vi "extraeIO.vi"(8 "error in TCP":errorcluster, 10 "path":path, 11 "connection IDin":refnum<k5>) -> (0 "error out TCP":errorcluster, 1 "output Controls":cluster{"name":string, "type desc":i16[]}[](array[cluster]), 2 "output Indicators":cluster{"name":string, "type desc":i16[]}[](array[cluster]), 3 "connection ID out":refnum<k5>, 4 "it is ok?":bool, 5 "error out":errorcluster, 7 "vi reference":refnum<vi>)   [LabVIEW 2010]
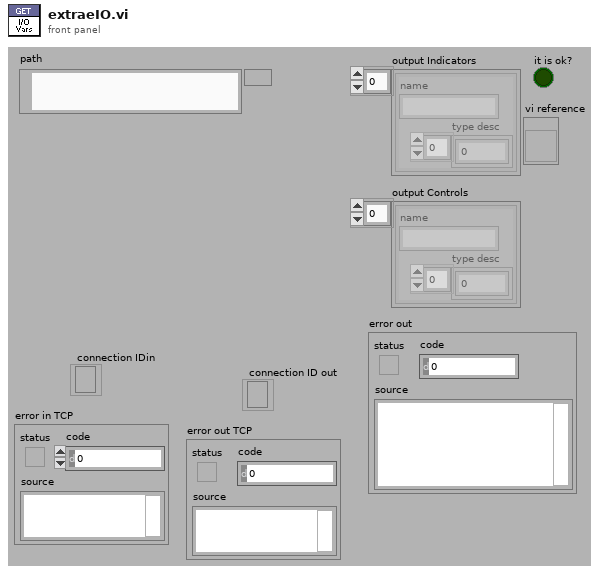
[diagram p1: front panel]
types:
  T1 = cluster{"name":string, "type desc":i16[], "flat data":string}[]
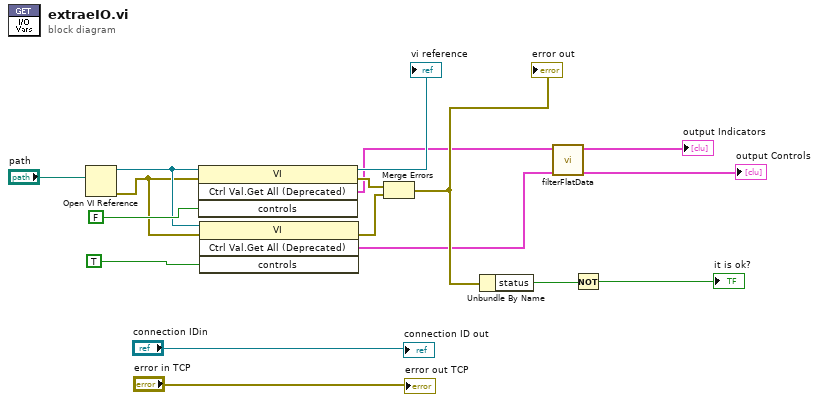
[diagram p0: block diagram]
diagram:
  n1 = Open VI Reference(vi path="path") -> (vi reference=w12:refnum<vi>, error out=w11:errorcluster)  [unwired: 2 in, 3 out]
  n2 = invoke class="VI" method="Ctrl Val.Get All (Deprecated)"(reference=w12, error in=w11, "controls"=FALSE ("Controls")) -> (reference out=→"vi reference":refnum<vi>, error out=w10:errorcluster, "Get All Control Values"=w8:T1)  [unwired: 1 in, 1 out]
  n3 = invoke class="VI" method="Ctrl Val.Get All (Deprecated)"(reference=w12, error in=w11, "controls"=TRUE ("Controls")) -> (error out=w9:errorcluster, "Get All Control Values"=w7:T1)  [unwired: 1 in, 2 out]
  n4 = Merge Errors(w10, w9) -> (w15:errorcluster)
  "error out" <- w15
  n5 = Unbundle By Name(w15) -> ("status"=w6:bool)
  n6 = call "filterFlatData.vi"("Data with flat data 2"=w7, "Data with flat data"=w8) -> ("Data without flat data 2"=→"output Controls":cluster{"name":string, "type desc":i16[]}[], "Data without flat data"=→"output Indicators":cluster{"name":string, "type desc":i16[]}[])  [unwired: 8 out]
  n7 = Not(x=w6) -> (.not. x?=→"it is ok?":bool)
  "connection ID out" <- "connection IDin"
  "error out TCP" <- "error in TCP"
